vi "Main.vi"() -> ()   [LabVIEW 2018]
uses:
  <vilib>/Waveform/WDTOps.llb/WDT Get Final Time Value DBL.vi
panel:
  out "State":dbl
  in  "For Debugging:":bool
  in  "Tab Control":T1(tab)
  out "Waveform Graph":waveform(dbl)[](graph)
  out "Tolerance":dbl
  out "Current (PV)":dbl
  in  "Abort":bool
  in  "Start":bool
  out "Status Feed":string
  in  "Save File(s) Location":path
  out "Estimated Time\nOf Completion":timestamp
  out "Start Time":timestamp
  out "DANGER":bool
  out "TTL Out (MV)":dbl
  out "Setpoint":dbl
  out "Temperature 5":dbl
  out "Temperature 3":dbl
  out "Temperature 4":dbl
  out "Temperature 2":dbl
  out "Measured Temperature":dbl
  out "Thermocouple 1":dbl(slide) scale=0.0..200.0
  out "Thermocouple 3":dbl(slide) scale=0.0..200.0
  out "Thermocouple 2":dbl(slide) scale=0.0..200.0
  out "Thermocouple 5":dbl(slide) scale=0.0..200.0
  out "Thermocouple 4":dbl(slide) scale=0.0..200.0
  in  "Read Channels":tag
  out "Resulting Setpoint Profile":cluster{"Time (s)":dbl, "Setpoint (Deg)":dbl}[](array[cluster])
  in  "RTO":dbl=25.0
  out "Current Room Temperature (Offset)":dbl
  in  "Gain Scheduling File Path":path
  in  "Temperature Schedule":T2(array[cluster])
  in  "Centigrade / Fahrenheit":bool
  in  "Set Schedules":bool
  in  "Clear Temp Schedule":bool
  in  "Select Default Process":bool
  in  "DefaulCycle":string(combo)
  out "Valid Process":bool
  in  "Debug (Don't Send Me a Message)":bool=TRUE
  in  "Body":string="Error"
  in  "Password":string
  in  "Email":string
  in  "Name of Experiment":string="LabVIEW Error"
  in  "Emergency Contact (Carrier)":enum16{"T-Mobile", "AT&T", "Verizon", "Sprint"}(ring)
  in  "Emergency Contact (phone number)":string
  in  "Temperature Tolerance (Degrees)":dbl=500.0
  in  "Max Rate Temperature":dbl=10.0
  in  "Min Temperature":dbl=10.0
  in  "Max Temperature":dbl=200.0
  out "Input Validated":bool
  out "Initialized":bool
  # "Temperature Readings"
  # "BLUE M SINGLEZONE FURNACE\nStable Build #1"
  # "^^^\nChange this in\nEquipment Properties"
  # "Temperature Settings"
  # "These represent the max allowable settings for the process. It is recommended that temperature limits should be set well within the safety limits of the equipment. Please allow generous safety margins!"
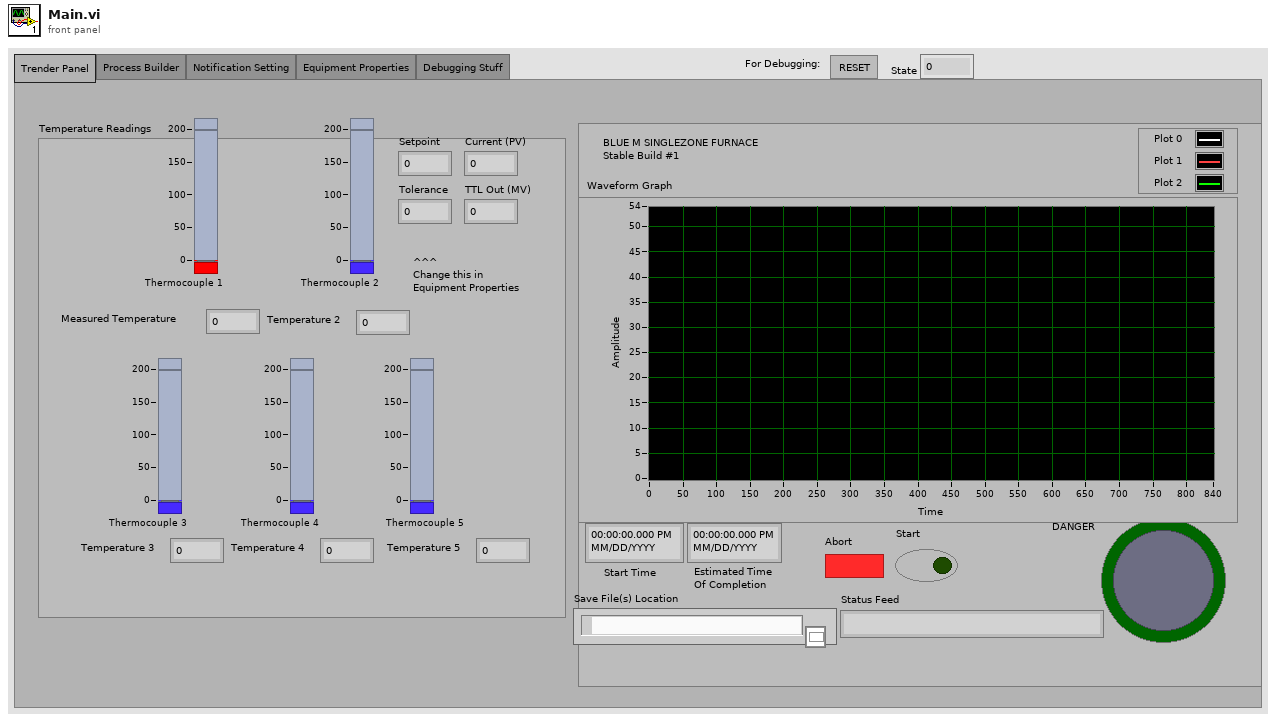
[diagram p1: front panel]
types:
  T1 = enum32{"Trender Panel", "Process Builder", "Notification Setting", "Equipment Properties", "Debugging Stuff"}
  T2 = cluster{"Duration (min)":dbl, "Ramp Rate (1/min)":dbl, "Data Frequency":dbl}[]
  T3 = cluster{"Max Temperature":dbl, "Min Temperature":dbl, "Max Rate Temperature":dbl}
  T4 = cluster{"time (s)":dbl, "setpoint ":dbl, "frequency":dbl}[]
  T5 = cluster{"Max Temperature":dbl, "Min Temperature":dbl}
  T6 = cluster{"Values Array":dbl[], "Timestamp Array":timestamp[]}[]
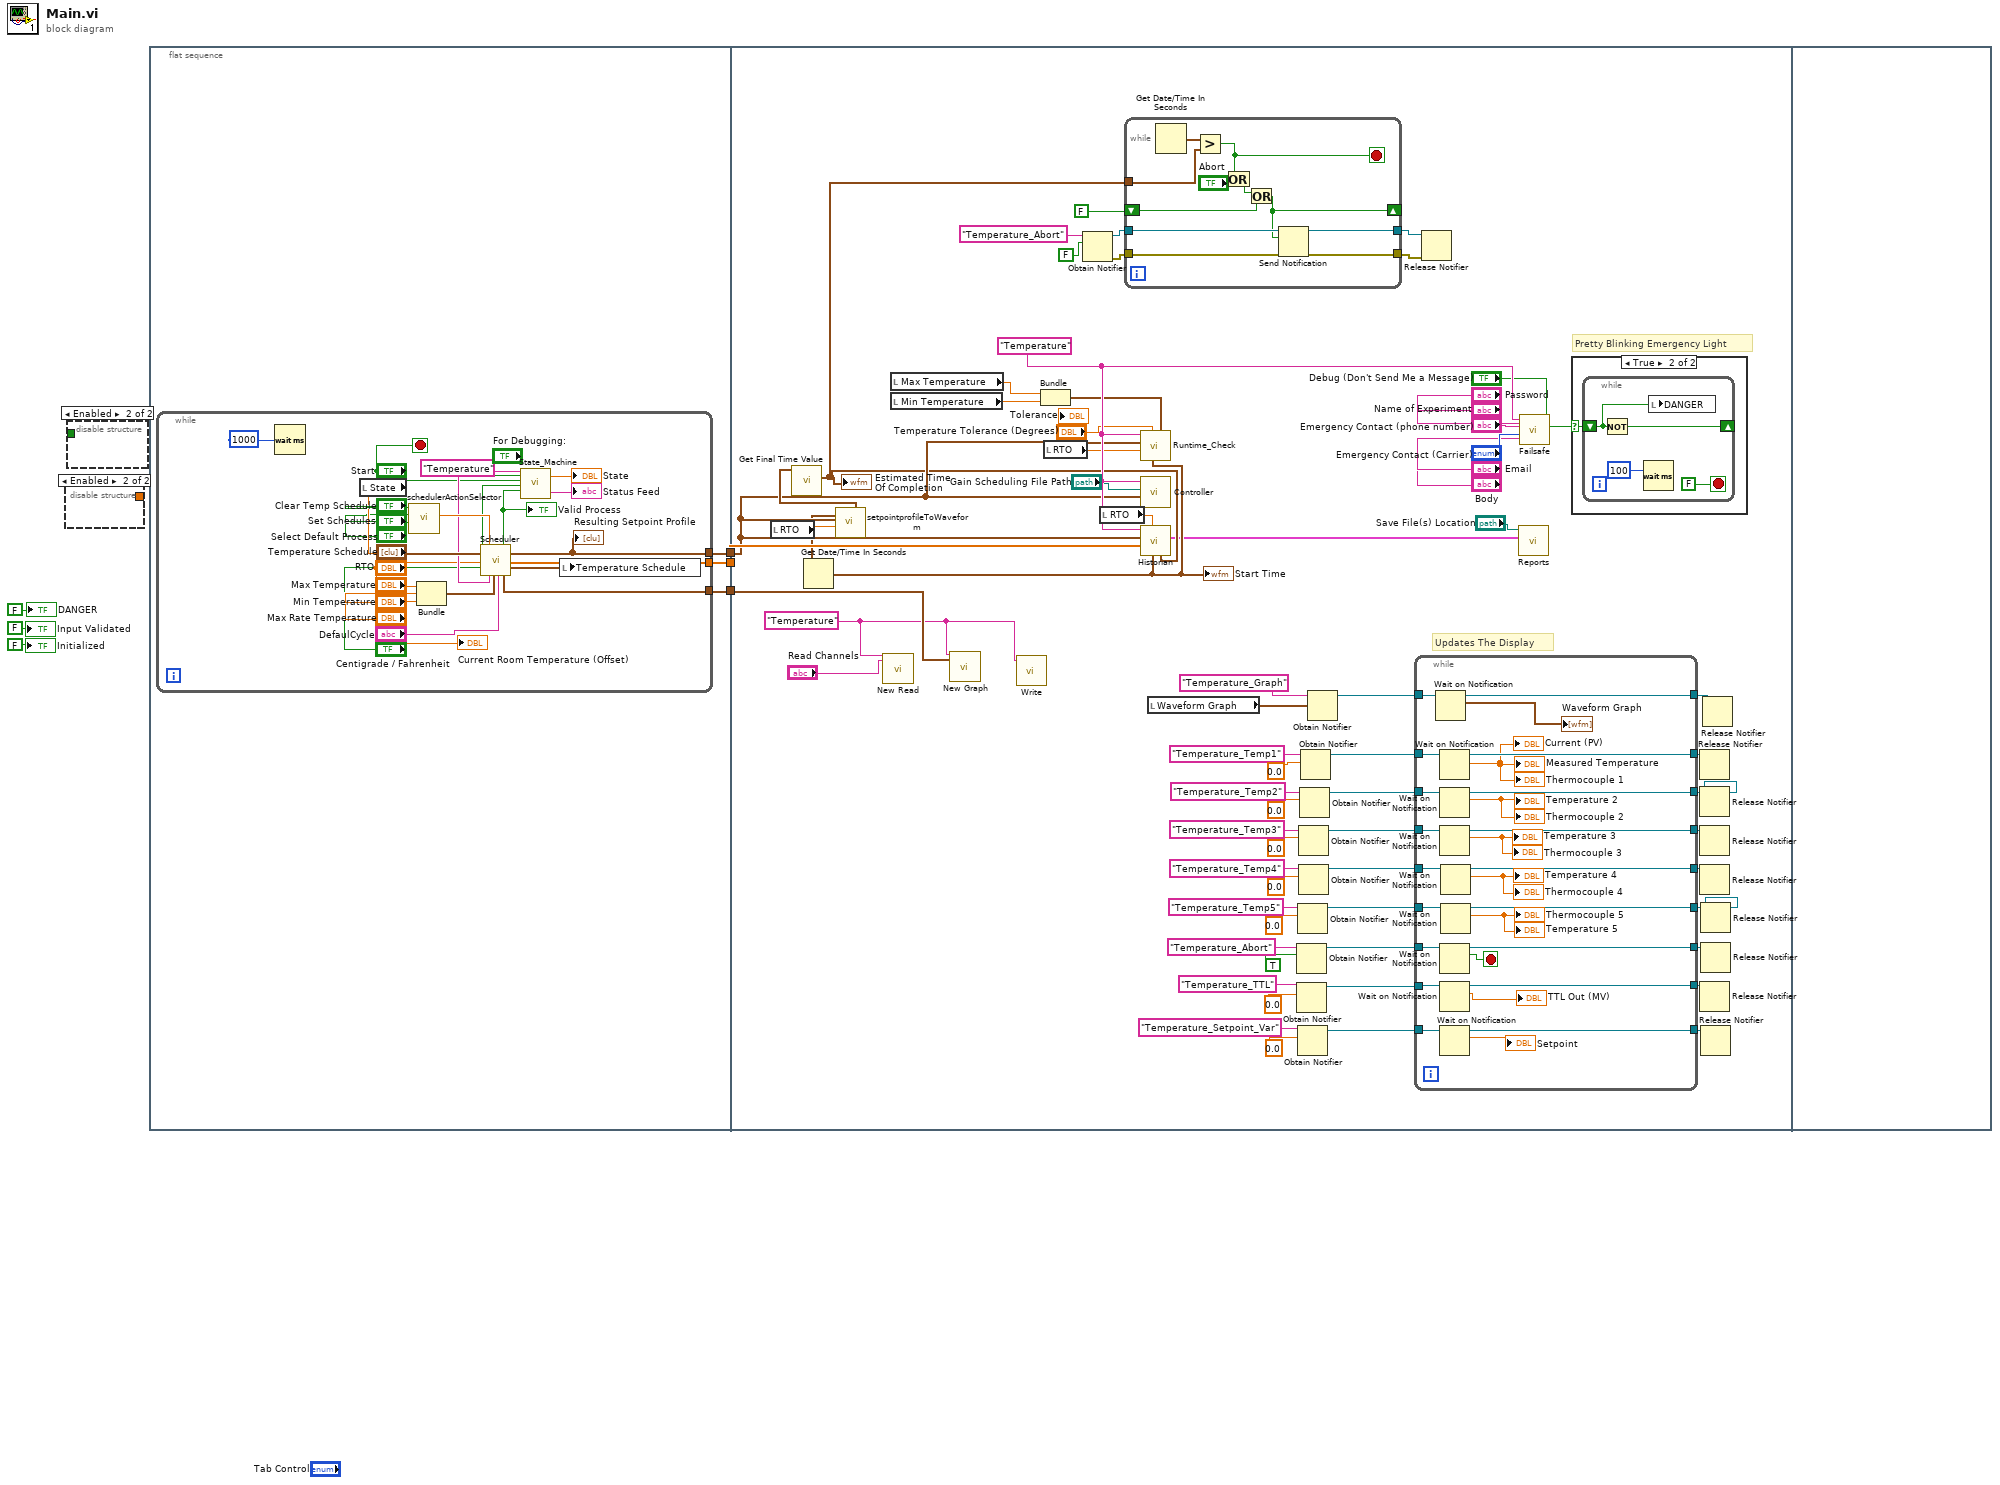
[diagram p0: block diagram]
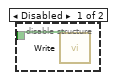
[diagram p2: hidden frame]
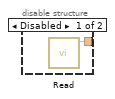
[diagram p3: hidden frame]
diagram:
  n1 = disable-structure shown="Enabled" {
    disable-tunnel: [w7 _] -> _
    frame Disabled {
      n2 = call "Read.vi"() -> (3:w7)  [unwired: 4 in, 7 out]
    }
    frame Enabled {
    }
  }
  n3 = disable-structure shown="Enabled" {
    disable-tunnel: _ -> [w8 _]
    frame Disabled {
      n4 = call "Write.vi"("Process_REF"=w8) -> ()  [unwired: 10 in, 1 out]
    }
    frame Enabled {
    }
  }
  n5 = flat-sequence {
    tunnel: [w11] -> w4
    tunnel: [w10] -> w3
    tunnel: [w9] -> w1
    tunnel: w4 -> [w105]
    tunnel: w3 -> [w97]
    tunnel: w1 -> [w39]
    frame #0 {
      n6 = while {
        tunnel: [w18] -> w11
        tunnel: [w13] -> w10
        tunnel: [w12] -> w9
        stop <- "Start" stop-if-true
        w21 = "Temperature"
        n7 = Wait (ms)(milliseconds to wait=1000) -> ()  [unwired: 1 out]
        n8 = local read "State"() -> (w25:dbl)
        n9 = call "schedulerActionSelector.vi"("Read Default Schedule"="Select Default Process", "Update Scheduler"="Set Schedules", "Clear Scheduler"="Clear Temp Schedule") -> ("Scheduler Action"=w35:dbl)  [unwired: 8 in]
        n10 = Bundle("Max Temperature"="Max Temperature", "Min Temperature"="Min Temperature", "Max Rate Temperature"="Max Rate Temperature") -> (w15:T3)  [unwired: 1 in]
        n11 = call "Scheduler.vi"("RampRates"="Temperature Schedule", "Room Temperature"="RTO", "CentigradeToFahrenheit"="Centigrade / Fahrenheit", "Action"=w35, "Process_REF"=w21, "State"=w25, "Machine Settings"=w15, "Read File"="DefaulCycle") -> ("Initialized"=w32:bool, "Is Valid Schedule"=w16:bool, "Waveform"=w12:waveform(dbl), "Setpoint Profile"=w13:cluster{"Time (s)":dbl, "setpoint (C)":dbl}[], "Sampling Rates"=w18:dbl[], "New RampRates"=w29:T4)  [unwired: 4 in, 2 out]
        "Valid Process" <- w16
        "Resulting Setpoint Profile" <- w13
        n12 = call "State_Machine.vi"("Process_REF"=w21, "Start Process"="Start", "Initialized"=w32, "Input Validated"=w16, "Reset"="For Debugging:") -> ("State"=→"State":dbl, "State String"=→"Status Feed":string)  [unwired: 11 in, 2 out]
        n13 = local write "Temperature Schedule"(w29) -> ()
        "Current Room Temperature (Offset)" <- "RTO"
      }
    }
    frame #1 {
      w38 = "Temperature"
      w99 = "Temperature"
      # "Pretty Blinking Emergency Light"
      # "Updates The Display"
      n14 = local read "RTO"() -> (w55:dbl)
      n15 = Get Date/Time In Seconds() -> (seconds since 1Jan1904=w54:timestamp)
      "Start Time" <- w54
      n16 = call "setpointprofileToWaveform.vi"("Start Time"=w54, "Room Temp Offset"=w55, "setpoint profile"=w97) -> ("Waveform"=w106:waveform(dbl))  [unwired: 8 in]
      n17 = call-poly <vilib>:"Get Final Time Value.vi"("waveform in"=w106) -> ("tf"=w51:timestamp)  [unwired: 8 in, 2 out]
      "Estimated Time\nOf Completion" <- w51
      n18 = call "New Read.vi"("Process_REF"=w38, "physical channels"="Read Channels") -> ()  [unwired: 26 in]
      n19 = local read "Max Temperature"() -> (w95:dbl)
      n20 = local read "Min Temperature"() -> (w94:dbl)
      n21 = call "New Graph.vi"("Process_REF"=w38, "Waveform"=w39) -> ()  [unwired: 26 in]
      n22 = call "Write.vi"("Process_REF"=w38) -> ()  [unwired: 10 in, 1 out]
      n23 = Bundle("Max Temperature"=w95, "Min Temperature"=w94) -> (w96:T5)  [unwired: 1 in]
      n24 = local read "RTO"() -> (w57:dbl)
      n25 = Obtain Notifier(name (unnamed)="Temperature_Abort", notification data type=FALSE) -> (notifier out=w52:refnum<notifier>, error out=w48:errorcluster)  [unwired: 2 in, 1 out]
      n26 = local read "RTO"() -> (w56:dbl)
      n27 = while {
        tunnel: w52 -> [w117]
        tunnel: w51 -> [w111]
        tunnel: [w116] -> w49
        tunnel: w48 -> [w115]
        tunnel: [w114] -> w47
        shift-right: [w109] -> _
        shift-left: FALSE -> [w108]
        stop <- w107 stop-if-true
        n28 = Get Date/Time In Seconds() -> (seconds since 1Jan1904=w112:timestamp)
        n29 = Greater?(x=w112, y=w111) -> (0:w107:bool)
        n30 = Or(x=w107, y="Abort") -> (x .or. y?=w110:bool)
        n31 = Or(x=w110, y=w108) -> (x .or. y?=w109:bool)
        n32 = Send Notification(notification=w109, notifier=w117, error in (no error)=w115) -> (notifier out=w116:refnum<notifier>, error out=w114:errorcluster)
      }
      n33 = call "Runtime_Check.vi"("Machine Settings"=w96, "Initial Timestamp"=w54, "Tolerance"="Temperature Tolerance (Degrees)", "Initial Value"=w57, "setpoint profile"=w97, "Process_REF"=w99) -> ()  [unwired: 2 in, 3 out]
      n34 = call "Controller.vi"("setpoint profile"=w97, "Gain Schedule Table Path"="Gain Scheduling File Path", "Process_REF"=w99) -> ()  [unwired: 6 in, 1 out]
      n35 = call "Historian.vi"("Time of Completion"=w51, "Initial Time Stamp"=w54, "Initial Value"=w56, "Sampling Rates"=w105, "setpoint profile"=w97, "Process_REF"=w99) -> ("Reports"=w44:T6)  [unwired: 4 in, 1 out]
      n36 = local read "Waveform Graph"() -> (w40:waveform(dbl)[])
      n37 = Obtain Notifier(name (unnamed)="Temperature_Abort", notification data type=TRUE) -> (notifier out=w71:refnum<notifier>)  [unwired: 2 in, 2 out]
      n38 = Obtain Notifier(name (unnamed)="Temperature_TTL", notification data type=0.0) -> (notifier out=w67:refnum<notifier>)  [unwired: 2 in, 2 out]
      n39 = Obtain Notifier(name (unnamed)="Temperature_Temp5", notification data type=0.0) -> (notifier out=w79:refnum<notifier>)  [unwired: 2 in, 2 out]
      n40 = Obtain Notifier(name (unnamed)="Temperature_Setpoint_Var", notification data type=0.0) -> (notifier out=w63:refnum<notifier>)  [unwired: 2 in, 2 out]
      n41 = Obtain Notifier(name (unnamed)="Temperature_Temp3", notification data type=0.0) -> (notifier out=w81:refnum<notifier>)  [unwired: 2 in, 2 out]
      n42 = Obtain Notifier(name (unnamed)="Temperature_Temp4", notification data type=0.0) -> (notifier out=w80:refnum<notifier>)  [unwired: 2 in, 2 out]
      n43 = Obtain Notifier(name (unnamed)="Temperature_Temp2", notification data type=0.0) -> (notifier out=w82:refnum<notifier>)  [unwired: 2 in, 2 out]
      n44 = Obtain Notifier(name (unnamed)="Temperature_Temp1", notification data type=0.0) -> (notifier out=w83:refnum<notifier>)  [unwired: 2 in, 2 out]
      n45 = Obtain Notifier(name (unnamed)="Temperature_Graph", notification data type=w40) -> (notifier out=w42:refnum<notifier>)  [unwired: 2 in, 2 out]
      n46 = while {
        tunnel: w83 -> [w145]
        tunnel: w82 -> [w146]
        tunnel: w81 -> [w147]
        tunnel: w80 -> [w148]
        tunnel: w79 -> [w149]
        tunnel: [w144] -> w78
        tunnel: [w143] -> w77
        tunnel: [w142] -> w76
        tunnel: [w141] -> w75
        tunnel: [w140] -> w74
        tunnel: w71 -> [w139]
        tunnel: [w138] -> w70
        tunnel: w67 -> [w136]
        tunnel: [w135] -> w66
        tunnel: w63 -> [w133]
        tunnel: [w132] -> w62
        tunnel: w42 -> [w125]
        tunnel: [w124] -> w41
        stop <- w137 stop-if-true
        n47 = Wait on Notification(notifier=w125) -> (notifier out=w124:refnum<notifier>, notification=→"Waveform Graph":waveform(dbl)[])  [unwired: 3 in, 2 out]
        n48 = Wait on Notification(notifier=w145) -> (notifier out=w144:refnum<notifier>, notification=→"Current (PV)" →"Thermocouple 1" →"Measured Temperature":dbl)  [unwired: 3 in, 2 out]
        n49 = Wait on Notification(notifier=w146) -> (notifier out=w143:refnum<notifier>, notification=→"Thermocouple 2" →"Temperature 2":dbl)  [unwired: 3 in, 2 out]
        n50 = Wait on Notification(notifier=w147) -> (notifier out=w142:refnum<notifier>, notification=→"Thermocouple 3" →"Temperature 3":dbl)  [unwired: 3 in, 2 out]
        n51 = Wait on Notification(notifier=w139) -> (notifier out=w138:refnum<notifier>, notification=w137:bool)  [unwired: 3 in, 2 out]
        n52 = Wait on Notification(notifier=w136) -> (notifier out=w135:refnum<notifier>, notification=→"TTL Out (MV)":dbl)  [unwired: 3 in, 2 out]
        n53 = Wait on Notification(notifier=w133) -> (notifier out=w132:refnum<notifier>, notification=→"Setpoint":dbl)  [unwired: 3 in, 2 out]
        n54 = Wait on Notification(notifier=w148) -> (notifier out=w141:refnum<notifier>, notification=→"Temperature 4" →"Thermocouple 4":dbl)  [unwired: 3 in, 2 out]
        n55 = Wait on Notification(notifier=w149) -> (notifier out=w140:refnum<notifier>, notification=→"Temperature 5" →"Thermocouple 5":dbl)  [unwired: 3 in, 2 out]
      }
      n56 = Release Notifier(notifier=w49, error in (no error)=w47) -> ()  [unwired: 1 in, 3 out]
      n57 = call "Reports.vi"("Reports"=w44, "Path In"="Save File(s) Location") -> ()  [unwired: 8 in]
      n58 = call "Failsafe.vi"("Debug(NoSend)"="Debug (Don't Send Me a Message)", "Body"="Body", "Password"="Password", "Email"="Email", "Name of Experiment"="Name of Experiment", "Emergency Contact (Carrier)"="Emergency Contact (Carrier)", "Emergency Contact (phone number)"="Emergency Contact (phone number)", "Process_REF"=w99) -> ("Danger"=w61:bool)  [unwired: 2 in, 1 out]
      n59 = case shown="True" w61 {
        selector: w61 -> [_ w118]
        frame False {
        }
        frame True {
          n60 = while {
            shift-right: [w120] -> _
            shift-left: w118 -> [w119]
            stop <- FALSE stop-if-true
            n61 = Not(x=w119) -> (.not. x?=w120:bool)
            n62 = Wait (ms)(milliseconds to wait=100) -> ()  [unwired: 1 out]
            n63 = local write "DANGER"(w119) -> ()
          }
        }
      }
      n64 = Release Notifier(notifier=w78) -> ()  [unwired: 2 in, 3 out]
      n65 = Release Notifier(notifier=w77) -> ()  [unwired: 2 in, 3 out]
      n66 = Release Notifier(notifier=w76) -> ()  [unwired: 2 in, 3 out]
      n67 = Release Notifier(notifier=w75) -> ()  [unwired: 2 in, 3 out]
      n68 = Release Notifier(notifier=w66) -> ()  [unwired: 2 in, 3 out]
      n69 = Release Notifier(notifier=w74) -> ()  [unwired: 2 in, 3 out]
      n70 = Release Notifier(notifier=w70) -> ()  [unwired: 2 in, 3 out]
      n71 = Release Notifier(notifier=w62) -> ()  [unwired: 2 in, 3 out]
      n72 = Release Notifier(notifier=w41) -> ()  [unwired: 2 in, 3 out]
      "Tolerance" <- "Temperature Tolerance (Degrees)"
    }
    frame #2 {
    }
  }
  "DANGER" <- FALSE
  "Initialized" <- FALSE
  "Input Validated" <- FALSE
